vi "CheckKinect.vi"(8 "error in":errorcluster) -> (0 "error out":errorcluster, 2 "Hot?":bool)   [LabVIEW 2013]
doc: "Uses the Kinect to signal to the robot whether the goal is hot or not. If hands are detected, the goal is hot. Otherwise, the goal is not hot."
uses:
  <vilib>/addons/Kinect/Skeleton Vertex Index.ctl
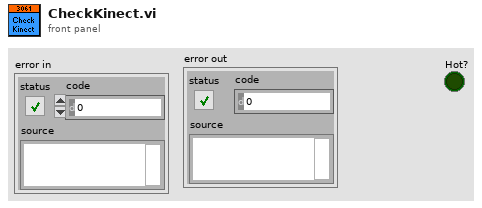
[diagram p1: front panel]
types:
  T1 = typedef "Skeleton Vertex Index.ctl" = i32
  T2 = typedef "SkeletonVertexTrackState.ctl" = enum32{"NotTracked", "Inferred", "Tracked"}
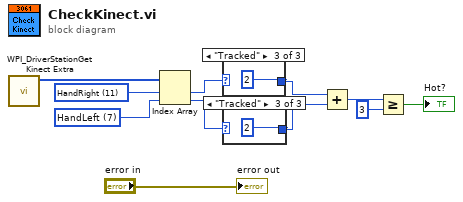
[diagram p0: block diagram]
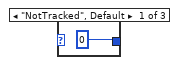
[diagram p2: hidden frame]
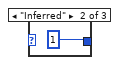
[diagram p3: hidden frame]
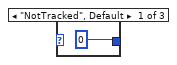
[diagram p4: hidden frame]
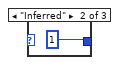
[diagram p5: hidden frame]
diagram:
  w9 = T1 7 items=["HipCenter", "Spine", "ShoulderCenter", "Head", "ShoulderLeft", "ElbowLeft", "WristLeft", "HandLeft", "ShoulderRight", "ElbowRight", "WristRight", "HandRight", "HipLeft", "KneeLeft", "AnkleLeft", "FootLeft", "HipRight", "KneeRight", "AnkleRight", "FootRight"] ("Skeleton Joints")
  w10 = T1 11 items=["HipCenter", "Spine", "ShoulderCenter", "Head", "ShoulderLeft", "ElbowLeft", "WristLeft", "HandLeft", "ShoulderRight", "ElbowRight", "WristRight", "HandRight", "HipLeft", "KneeLeft", "AnkleLeft", "FootLeft", "HipRight", "KneeRight", "AnkleRight", "FootRight"] ("Skeleton Joints")
  n1 = call <vilib>:"WPI_DriverStationGet Kinect Extra.vi"() -> ("Skeleton Tracking State"=w11:T2[])  [unwired: 7 in, 4 out]
  n2 = Index Array(array=w11, index #1=w10, index #2=w9) -> (element #1=w7:T2, element #2=w8:T2)
  n3 = case shown="\"Tracked\"" w7 {
    tunnel: [0 1 2] -> w6
    frame "NotTracked", Default {
    }
    frame "Inferred" {
    }
    frame "Tracked" {
    }
  }
  n4 = case shown="\"Tracked\"" w8 {
    tunnel: [0 1 2] -> w5
    frame "NotTracked", Default {
    }
    frame "Inferred" {
    }
    frame "Tracked" {
    }
  }
  n5 = Add(x=w6, y=w5) -> (x+y=w4:i32)
  n6 = Greater Or Equal?(x=w4, y=3) -> (x >= y?=→"Hot?":bool)
  "error out" <- "error in"
